vi "SetSMUSense.vi"(7 "SMU":T2, 8 "Error In":errorcluster, 10 "SMU Sense":T1, 11 "Keithley 2602 In":refnum<visa-resource-name>) -> (0 "Error Out":errorcluster, 3 "Keithley 2602 Out":refnum<visa-resource-name>)   [LabVIEW 2012, in "Keithley-2602.lvlib"]
uses:
  Keithley-2602.lvlib
  Controls/SMU.ctl
  Controls/SMUSense.ctl
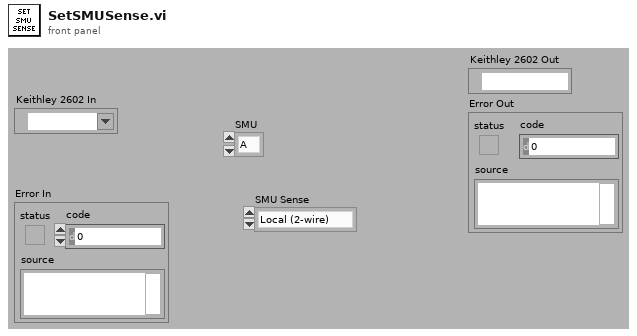
[diagram p1: front panel]
types:
  T1 = typedef "Keithley-2602.lvlib/SMUSense.ctl" = enum16{"Local (2-wire)", "Remote (4-wire)", "Calibration"}
  T2 = typedef "Keithley-2602.lvlib/SMU.ctl" = enum16{"A", "B"}
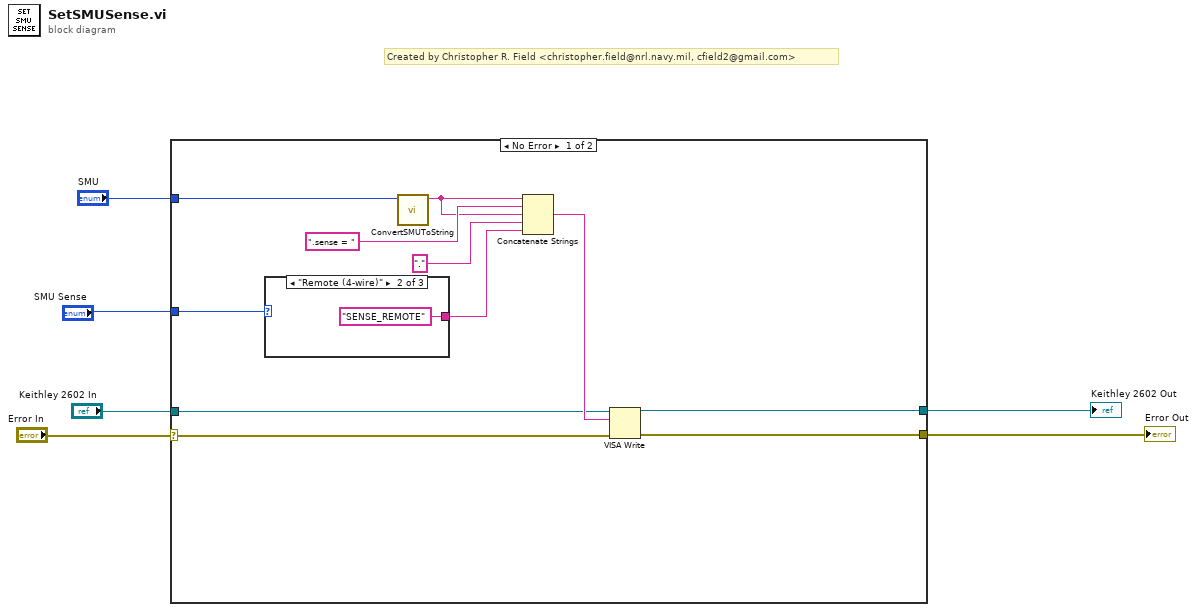
[diagram p0: block diagram]
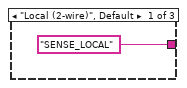
[diagram p2: hidden frame]
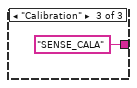
[diagram p3: hidden frame]
diagram:
  # "Created by Christopher R. Field <christopher.field@nrl.navy.mil, cfield2@gmail.com>"
  n1 = case shown="No Error" "Error In" {
    selector: "Error In" -> [w7 w21]
    tunnel: "Keithley 2602 In" -> [w12 w22]
    tunnel: [w11 w22] -> w5
    tunnel: [w10 w21] -> w4
    tunnel: "SMU" -> [w9 _]
    tunnel: "SMU Sense" -> [w8 _]
    frame No Error {
      n2 = case shown="\"Remote (4-wire)\"" w8 {
        tunnel: ["SENSE_LOCAL" "SENSE_REMOTE" "SENSE_CALA"] -> w14
        frame "Local (2-wire)", Default {
        }
        frame "Remote (4-wire)" {
        }
        frame "Calibration" {
        }
      }
      n3 = call "ConvertSMUToString.vi"("SMU"=w9) -> ("Channel"=w16:string)  [unwired: 10 in]
      n4 = Concatenate Strings(w16, ".sense = ", w16, "." ("string"), w14) -> (w13:string)
      n5 = VISA Write(VISA resource name=w12, write buffer=w13, error in (no error)=w7) -> (VISA resource name out=w11:refnum<visa-resource-name>, error out=w10:errorcluster)  [unwired: 1 out]
    }
    frame Error {
    }
  }
  "Keithley 2602 Out" <- w5
  "Error Out" <- w4
